vi "Build Item Tag.vi"(8 "error in":errorcluster, 10 "Parent Tag":string, 11 "LabVIEWItem in":refnum<class "LabVIEWItem.lvclass">) -> (0 "error out":errorcluster, 3 "LabVIEWItem out":refnum<class "LabVIEWItem.lvclass">)   [LabVIEW 2019, in "Panther Dashboard.lvlib" / "LabVIEWItem.lvclass"]
uses:
  LabVIEWItem.lvclass
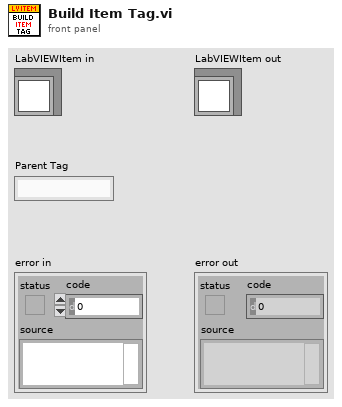
[diagram p1: front panel]
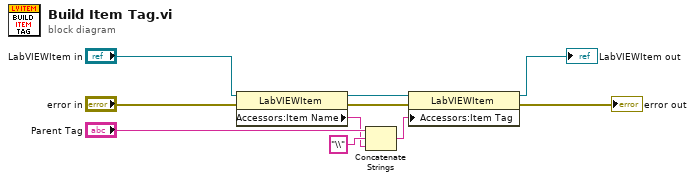
[diagram p0: block diagram]
diagram:
  n1 = property class="LabVIEWItem"(reference="LabVIEWItem in", error in="error in") -> (reference out=w2:refnum<class "LabVIEWItem.lvclass">, error out=w8:errorcluster, "Accessors:Item Name"=w1:string)
  n2 = Concatenate Strings("Parent Tag", "\\" ("string"), w1) -> (w4:string)
  n3 = property class="LabVIEWItem"(reference=w2, error in=w8, "Accessors:Item Tag"=w4) -> (reference out=→"LabVIEWItem out":refnum<class "LabVIEWItem.lvclass">, error out=→"error out":errorcluster)
